vi "Compile UEGO.vi"(8 "error in (no error)":errorcluster, 11 "Device Ref in":T2 format="%.0x") -> (0 "error out":errorcluster, 2 "UEGO Calibration Info":T1[](array[typedef]), 3 "Device Ref out":T2=18446744073709551615 format="%.0x")   [LabVIEW 2014, in "SLSC configuration System Explorer.lvlib"]
uses:
  SLSC configuration System Explorer.lvlib
  Shared/Constants.vi
  Shared/SLSC configuration Shared.lvlib
  <vilib>/NI Veristand/Custom Device API/Custom Device API.lvlib
  <vilib>/NI Veristand/Custom Device API/Get Item Property (U32).vi
  <vilib>/NI Veristand/Custom Device Tools/Custom Device Utility Library/Custom Device Utility Library.lvlib
  Type Defs/UEGO Compile Info.ctl
  <vilib>/NI Veristand/Custom Device API/Get Item Property (String).vi
  <vilib>/NI Veristand/Custom Device API/Custom Device Item Ref.ctl
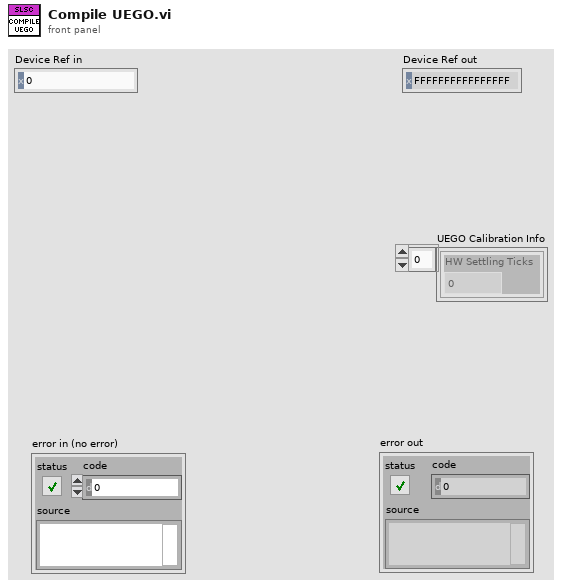
[diagram p1: front panel]
types:
  T1 = typedef "SLSC configuration Shared.lvlib/UEGO Compile Info.ctl" = cluster{"HW Settling Ticks":u32}
  T2 = typedef "Custom Device API.lvlib/Custom Device Item Ref.ctl" = u64
  T3 = typedef "SLSC configuration Shared.lvlib/Card Position.ctl" = cluster{"Rack #":u8, "Slot #":T4}
  T4 = typedef "SLSC configuration Shared.lvlib/Slot #.ctl" = u8
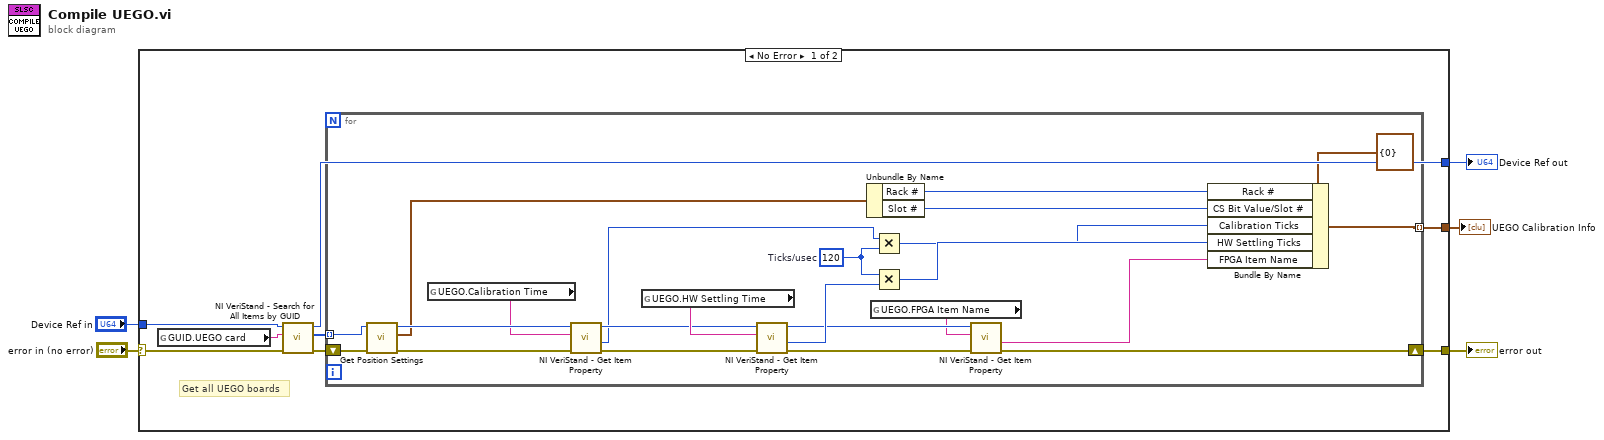
[diagram p0: block diagram]
diagram:
  n1 = case shown="No Error" "error in (no error)" {
    selector: "error in (no error)" -> [w12 w38]
    tunnel: [w9 w38] -> w2
    tunnel: [w8 _] -> w1
    tunnel: "Device Ref in" -> [w7 w37]
    tunnel: [w6 w37] -> w3
    frame No Error {
      # "Get all UEGO boards"
      n2 = global read "Constants.vi" "GUID.UEGO card"() -> (w13:string)
      n3 = call <vilib>:"NI VeriStand - Search for All Items by GUID.vi"("error in"=w12, "Item GUID"=w13, "Section Ref in"=w7) -> ("error out"=w11:errorcluster, "Item Refs"=w10:T2[], "Section Ref out"=w6:T2)  [unwired: 5 in, 1 out]
      n4 = for {
        tunnel: w10 -> [w22] mode=indexing
        shift-right: [w16] -> w9
        shift-left: w11 -> [w21]
        tunnel: [w20] -> w8 mode=indexing
        w35 = u32 120  # Ticks/usec
        n5 = call "Get Position Settings.vi"("error in (no error)"=w21, "Item Ref in"=w22) -> ("error out"=w28:errorcluster, "Card Position"=w23:T3, "Item Ref out"=w27:T2)  [unwired: 7 in]
        n6 = global read "Constants.vi" "UEGO.Calibration Time"() -> (w26:string)
        n7 = call-poly <vilib>:"NI VeriStand - Get Item Property.vi"("error in (no error)"=w28, "Property Name"=w26, "Item Ref in"=w27) -> ("error out"=w31:errorcluster, "Value"=w29:u32, "Item Ref out"=w32:T2)  [unwired: 5 in, 1 out]
        n8 = global read "Constants.vi" "UEGO.HW Settling Time"() -> (w33:string)
        n9 = call-poly <vilib>:"NI VeriStand - Get Item Property.vi"("error in (no error)"=w31, "Property Name"=w33, "Item Ref in"=w32) -> ("error out"=w18:errorcluster, "Value"=w34:u32, "Item Ref out"=w17:T2)  [unwired: 5 in, 1 out]
        n10 = Unbundle By Name(w23) -> ("Rack #"=w24:u8, "Slot #"=w25:T4)
        n11 = global read "Constants.vi" "UEGO.FPGA Item Name"() -> (w15:string)
        n12 = Multiply(x=w29, y=w35) -> (x*y=w30:u32)
        n13 = Multiply(x=w35, y=w34) -> (x*y=w36:u32)
        n14 = call-poly <vilib>:"NI VeriStand - Get Item Property.vi"("error in (no error)"=w18, "Property Name"=w15, "Item Ref in"=w17) -> ("error out"=w16:errorcluster, "Value"=w14:string)  [unwired: 5 in, 2 out]
        n15 = Bundle By Name(cluster=T1 {"HW Settling Ticks"=0} ("UEGO Compiled Info"), "Rack #"=w24, "CS Bit Value/Slot #"=w25, "Calibration Ticks"=w30, "HW Settling Ticks"=w36, "FPGA Item Name"=w14) -> (w20:T1)
      }
    }
    frame Error {
    }
  }
  "error out" <- w2
  "Device Ref out" <- w3
  "UEGO Calibration Info" <- w1
